vi "Const Language Default.vi"() -> (3 "UI Descriptions":T1={"Title"={"Frame Num"={"Name"="Frame Num", "Tip"=""}, "Name"={"Name"="Name", "Tip"=""}}, "Frame Basic"={"pic"={"Name"="pic", "Tip"=""}, "state"={"Name"="state", "Tip"=""}, "wait"={"Name"="wait", "Tip"=""}, "next"={"Name"="next", "Tip"=""}, "dvx"={"Name"="dvx", "Tip"=""}, "dvy"={"Name"="dvy", "Tip"=""}, "dvz"={"Name"="dvz", "Tip"=""}, "centerx"={"Name"="centerx", "Tip"=""}, "centery"={"Name"="centery", "Tip"=""}, "sound"={"Name"="sound", "Tip"=""}}, "Frame Skill"={"mp"={"Name"="mp", "Tip"=""}, "hit_a"={"Name"="hit_a", "Tip"=""}, "hit_d"={"Name"="hit_d", "Tip"=""}, "hit_j"={"Name"="hit_j", "Tip"=""}, "hit_Fa"={"Name"="hit_Fa", "Tip"=""}, "hit_Ua"={"Name"="hit_Ua", "Tip"=""}, "hit_Da"={"Name"="hit_Da", "Tip"=""}, "hit_Fj"={"Name"="hit_Fj", "Tip"=""}, "hit_Uj"={"Name"="hit_Uj", "Tip"=""}, "hit_Dj"={"Name"="hit_Dj", "Tip"=""}, "hit_ja"={"Name"="hit_ja", "Tip"=""}}, "bp"={"x"={"Name"="x", "Tip"=""}, "y"={"Name"="y", "Tip"=""}}, "w"={"kind"={"Name"="kind", "Tip"=""}, "x"={"Name"="x", "Tip"=""}, "y"={"Name"="y", "Tip"=""}, "weaponact"={"Name"="weaponact", "Tip"=""}, "cover"={"Name"="cover", "Tip"=""}, "dvx"={"Name"="dvx", "Tip"=""}, "dvy"={"Name"="dvy", "Tip"=""}, "dvz"={"Name"="dvz", "Tip"=""}, "attacking"={"Name"="attacking", "Tip"=""}}, "b"={"kind"={"Name"="kind", "Tip"=""}, "x"={"Name"="x", "Tip"=""}, "y"={"Name"="y", "Tip"=""}, "w"={"Name"="w", "Tip"=""}, "h"={"Name"="h", "Tip"=""}}, "i"={"kind"={"Name"="kind", "Tip"=""}, "x"={"Name"="x", "Tip"=""}, "y"={"Name"="y", "Tip"=""}, "w"={"Name"="w", "Tip"=""}, "h"={"Name"="h", "Tip"=""}, "zwidth"={"Name"="zwidth", "Tip"=""}, "dvx"={"Name"="dvx", "Tip"=""}, "dvy"={"Name"="dvy", "Tip"=""}, "dvz"={"Name"="dvz", "Tip"=""}, "fall"={"Name"="fall", "Tip"=""}, "arest"={"Name"="arest", "Tip"=""}, "vrest"={"Name"="vrest", "Tip"=""}, "bdefend"={"Name"="bdefend", "Tip"=""}, "injury"={"Name"="injury", "Tip"=""}, "effect"={"Name"="effect", "Tip"=""}, "catchingact 1"={"Name"="catchingact 1", "Tip"=""}, "catchingact 2"={"Name"="catchingact 2", "Tip"=""}, "caughtact 1"={"Name"="caughtact 1", "Tip"=""}, "caughtact 2"={"Name"="caughtact 2", "Tip"=""}}, "o"={"kind"={"Name"="kind", "Tip"=""}, "x"={"Name"="x", "Tip"=""}, "y"={"Name"="y", "Tip"=""}, "action"={"Name"="action", "Tip"=""}, "dvx"={"Name"="dvx", "Tip"=""}, "dvy"={"Name"="dvy", "Tip"=""}, "dvz"={"Name"="dvz", "Tip"=""}, "oid"={"Name"="oid", "Tip"=""}, "facing"={"Name"="facing", "Tip"=""}}, "c"={"kind"={"Name"="kind", "Tip"=""}, "x"={"Name"="x", "Tip"=""}, "y"={"Name"="y", "Tip"=""}, "injury"={"Name"="injury", "Tip"=""}, "cover"={"Name"="cover", "Tip"=""}, "vaction"={"Name"="vaction", "Tip"=""}, "aaction"={"Name"="aaction", "Tip"=""}, "taction"={"Name"="taction", "Tip"=""}, "hurtable"={"Name"="hurtable", "Tip"=""}, "decrease"={"Name"="decrease", "Tip"=""}, "fronthurtact"={"Name"="fronthurtact", "Tip"=""}, "backhurtact"={"Name"="backhurtact", "Tip"=""}, "throwvx"={"Name"="throwvx", "Tip"=""}, "throwvy"={"Name"="throwvy", "Tip"=""}, "throwvz"={"Name"="throwvz", "Tip"=""}, "throwinjury"={"Name"="throwinjury", "Tip"=""}, "dircontrol"={"Name"="dircontrol", "Tip"=""}}})   [LabVIEW 2018, in "LF2R IDE.lvlib" / "LF2R IDE.lvclass"]
uses:
  LF2R IDE.lvclass
  Const UI Description Setting.ctl
  Const UI Desc Frame Title.ctl
  Const UI Property.ctl
  Const UI Desc Frame Basic.ctl
  Const UI Desc Frame Skill.ctl
  Const UI Desc Frame bp.ctl
  Const UI Desc Frame w.ctl
  Const UI Desc Frame b.ctl
  Const UI Desc Frame i.ctl
  Const UI Desc Frame o.ctl
  Const UI Desc Frame c.ctl
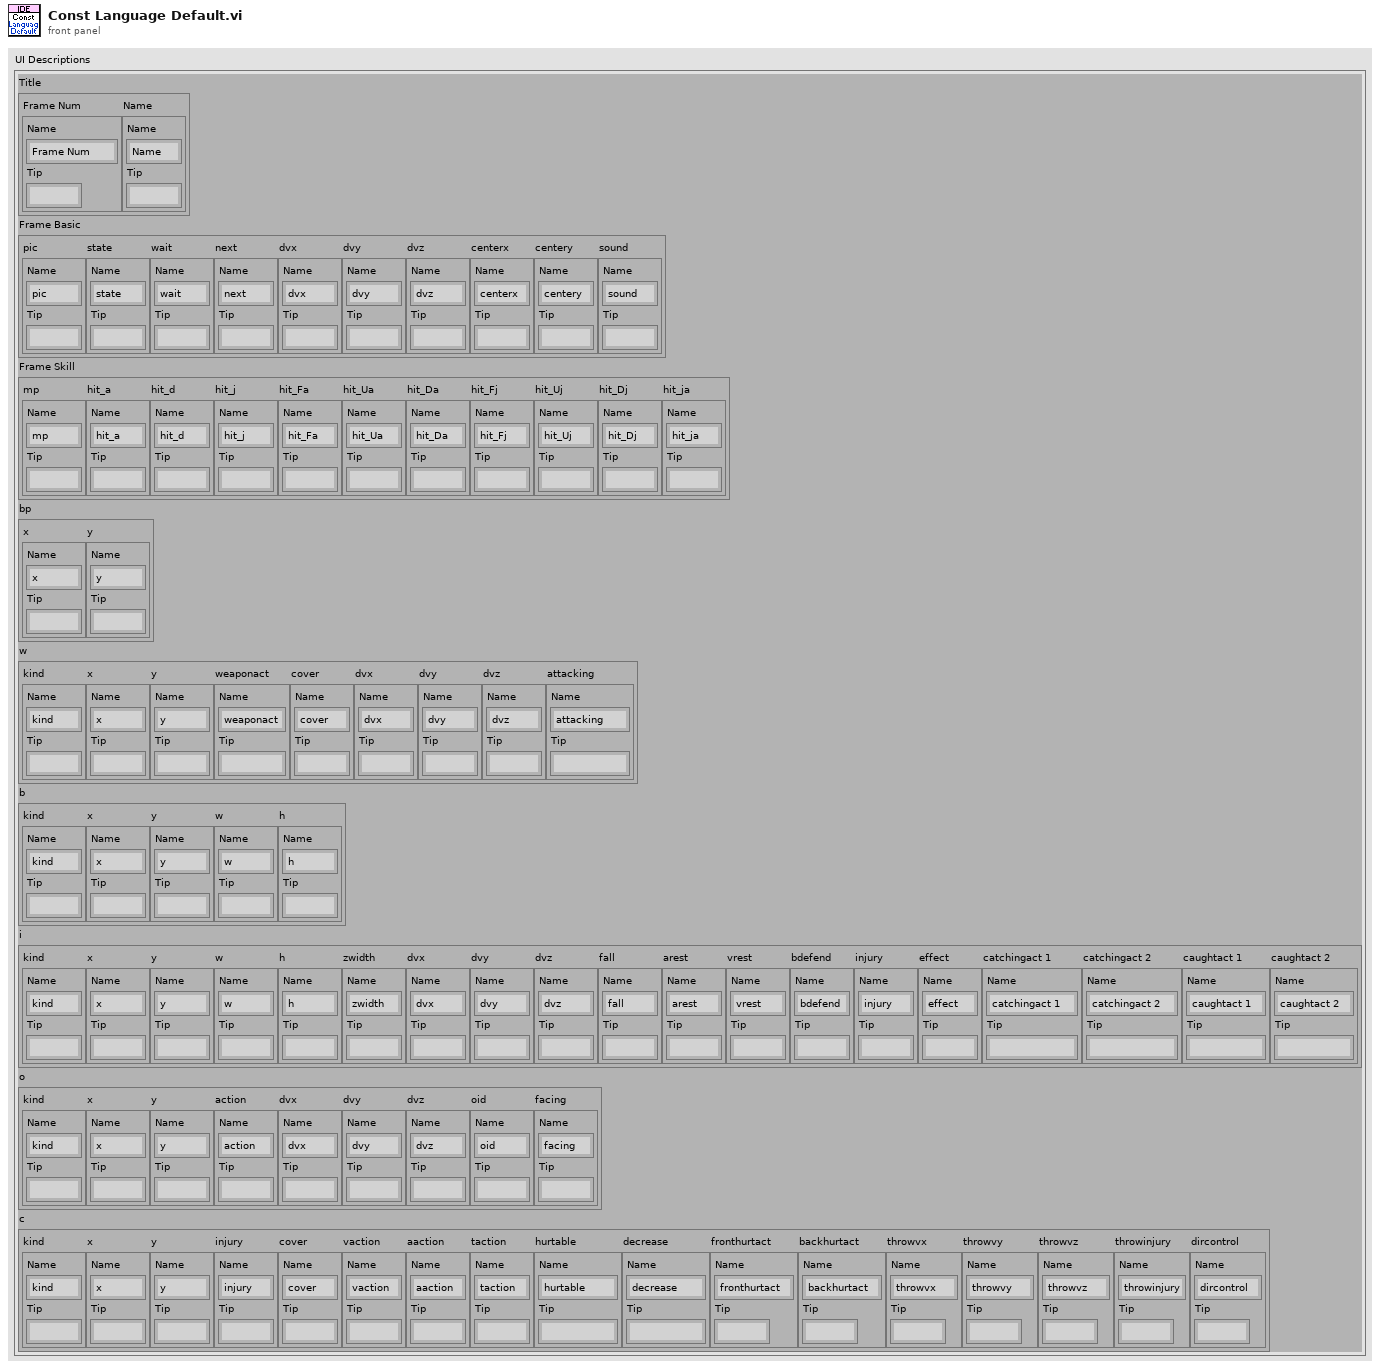
[diagram p1: front panel]
types:
  T1 = typedef "LF2R IDE.lvlib/LF2R IDE.lvclass/Const UI Description Setting.ctl" = cluster{"Title":T2, "Frame Basic":T4, "Frame Skill":T5, "bp":T6, "w":T7, "b":T8, "i":T9, "o":T10, "c":T11}
  T2 = typedef "LF2R IDE.lvlib/LF2R IDE.lvclass/Const UI Desc Frame Title.ctl" = cluster{"Frame Num":T3, "Name":T3}
  T3 = typedef "LF2R IDE.lvlib/LF2R IDE.lvclass/Const UI Property.ctl" = cluster{"Name":string, "Tip":string}
  T4 = typedef "LF2R IDE.lvlib/LF2R IDE.lvclass/Const UI Desc Frame Basic.ctl" = cluster{"pic":T3, "state":T3, "wait":T3, "next":T3, "dvx":T3, "dvy":T3, "dvz":T3, "centerx":T3, "centery":T3, "sound":T3}
  T5 = typedef "LF2R IDE.lvlib/LF2R IDE.lvclass/Const UI Desc Frame Skill.ctl" = cluster{"mp":T3, "hit_a":T3, "hit_d":T3, "hit_j":T3, "hit_Fa":T3, "hit_Ua":T3, "hit_Da":T3, "hit_Fj":T3, "hit_Uj":T3, "hit_Dj":T3, "hit_ja":T3}
  T6 = typedef "LF2R IDE.lvlib/LF2R IDE.lvclass/Const UI Desc Frame bp.ctl" = cluster{"x":T3, "y":T3}
  T7 = typedef "LF2R IDE.lvlib/LF2R IDE.lvclass/Const UI Desc Frame w.ctl" = cluster{"kind":T3, "x":T3, "y":T3, "weaponact":T3, "cover":T3, "dvx":T3, "dvy":T3, "dvz":T3, "attacking":T3}
  T8 = typedef "LF2R IDE.lvlib/LF2R IDE.lvclass/Const UI Desc Frame b.ctl" = cluster{"kind":T3, "x":T3, "y":T3, "w":T3, "h":T3}
  T9 = typedef "LF2R IDE.lvlib/LF2R IDE.lvclass/Const UI Desc Frame i.ctl" = cluster{"kind":T3, "x":T3, "y":T3, "w":T3, "h":T3, "zwidth":T3, "dvx":T3, "dvy":T3, "dvz":T3, "fall":T3, "arest":T3, "vrest":T3, "bdefend":T3, "injury":T3, "effect":T3, "catchingact 1":T3, "catchingact 2":T3, "caughtact 1":T3, "caughtact 2":T3}
  T10 = typedef "LF2R IDE.lvlib/LF2R IDE.lvclass/Const UI Desc Frame o.ctl" = cluster{"kind":T3, "x":T3, "y":T3, "action":T3, "dvx":T3, "dvy":T3, "dvz":T3, "oid":T3, "facing":T3}
  T11 = typedef "LF2R IDE.lvlib/LF2R IDE.lvclass/Const UI Desc Frame c.ctl" = cluster{"kind":T3, "x":T3, "y":T3, "injury":T3, "cover":T3, "vaction":T3, "aaction":T3, "taction":T3, "hurtable":T3, "decrease":T3, "fronthurtact":T3, "backhurtact":T3, "throwvx":T3, "throwvy":T3, "throwvz":T3, "throwinjury":T3, "dircontrol":T3}
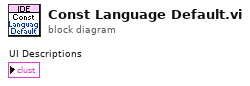
[diagram p0: block diagram]
diagram:
